vi "enable_all_buttons.vi"(0 "array":refnum<vi>[](array[refnum])) -> ()   [LabVIEW 2010]
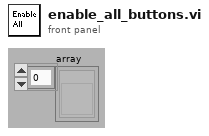
[diagram p1: front panel]
types:
  T1 = cluster{"array[0]":refnum<vi>, "array[1]":refnum<vi>, "array[2]":refnum<vi>, "array[3]":refnum<vi>, "array[4]":refnum<vi>, "array[5]":refnum<vi>}
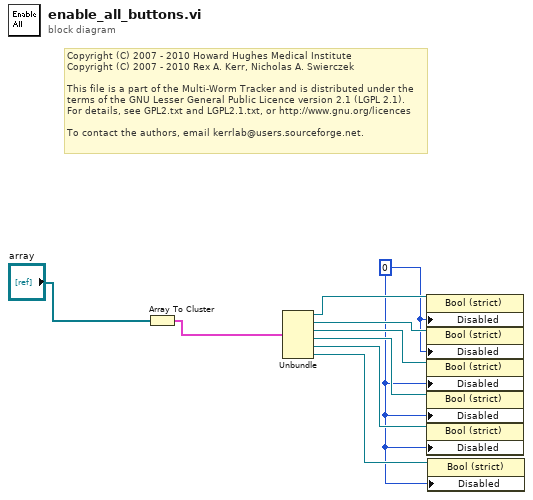
[diagram p0: block diagram]
diagram:
  w1 = u8 0 ("Disabled")
  # "Copyright (C) 2007 - 2010 Howard Hughes Medical Institute\nCopyright (C) 2007 - 2010 Rex A. Kerr, Nicholas A. Swierczek\n \nThis file is a part of the Multi-Worm Tracker and is distributed under the\nterms of the GNU Lesser General Public Licence version 2.1 (LGPL 2.1).\nFor details, see GPL2.txt and LGPL2.1.txt, or http://www.gnu.org/licences\n \nTo contact the authors, email kerrlab@users.sourceforge.net."
  n1 = Array To Cluster(array="array") -> (cluster=w4:T1)
  n2 = Unbundle(w4) -> ("array[0]"=w9:refnum<vi>, "array[1]"=w8:refnum<vi>, "array[2]"=w7:refnum<vi>, "array[3]"=w6:refnum<vi>, "array[4]"=w5:refnum<vi>, "array[5]"=w2:refnum<vi>)
  n3 = property class="Bool (strict)"(reference=w9, "Disabled"=w1) -> ()  [unwired: 1 in, 2 out]
  n4 = property class="Bool (strict)"(reference=w8, "Disabled"=w1) -> ()  [unwired: 1 in, 2 out]
  n5 = property class="Bool (strict)"(reference=w7, "Disabled"=w1) -> ()  [unwired: 1 in, 2 out]
  n6 = property class="Bool (strict)"(reference=w6, "Disabled"=w1) -> ()  [unwired: 1 in, 2 out]
  n7 = property class="Bool (strict)"(reference=w5, "Disabled"=w1) -> ()  [unwired: 1 in, 2 out]
  n8 = property class="Bool (strict)"(reference=w2, "Disabled"=w1) -> ()  [unwired: 1 in, 2 out]
